vi "generateTestStaticWfms.vi"(11 "Static Values":dbl[](array[numeric])) -> (3 "waveforms":waveform(dbl)[](array[waveform]))   [LabVIEW 2017]
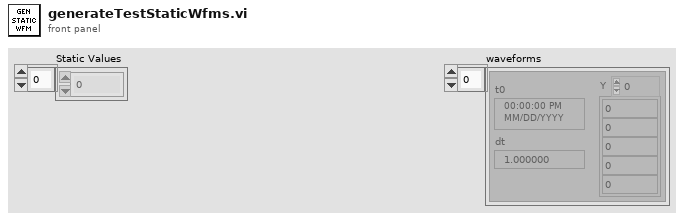
[diagram p1: front panel]
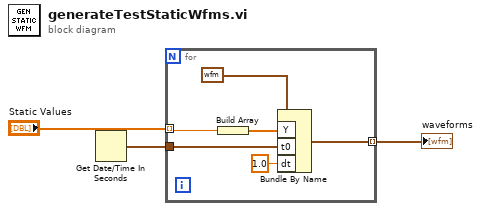
[diagram p0: block diagram]
diagram:
  n1 = Get Date/Time In Seconds() -> (seconds since 1Jan1904=w2:timestamp)
  n2 = for {
    tunnel: "Static Values" -> [w8] mode=indexing
    tunnel: w2 -> [w6]
    tunnel: [w4] -> w1 mode=indexing
    n3 = Build Array(w8) -> (w7:dbl[])
    n4 = Bundle By Name(cluster=waveform(dbl) {"t0"=timestamp(0 s since 1904-01-01), "dt"=1.0, "Y"=[]} ("Waveform"), "Y"=w7, "t0"=w6, "dt"=1.0) -> (w4:waveform(dbl))
  }
  "waveforms" <- w1
